vi "居中.vi"(8 "错误输入（无错误）":errorcluster, 11 "引用输入":refnum<vi>) -> (0 "错误输出":errorcluster, 3 "引用输出":refnum<vi>)   [LabVIEW 8.6, in "窗口操作.lvlib"]
doc: "<B>引用输入：</B>需要改变窗口的引用\n<B>引用输出：</B>需要改变窗口的引用输出\n\n编写者 ：曾嘉康\n编写时间：2014/12/12"
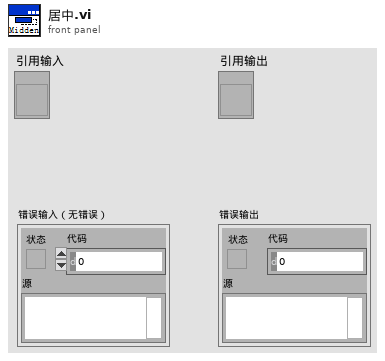
[diagram p1: front panel]
types:
  T1 = typedef "LVAllMonitorsDisplayTypeDef.ctl" = cluster{"Bounds":cluster{"Left":i16, "Top":i16, "Right":i16, "Bottom":i16}, "Depth":i16}[]
  T2 = typedef "LVRectTypeDef.ctl" = cluster{"Left":i16, "Top":i16, "Right":i16, "Bottom":i16}
  T3 = cluster{"Bounds":cluster{"Left":i16, "Top":i16, "Right":i16, "Bottom":i16}, "Depth":i16}
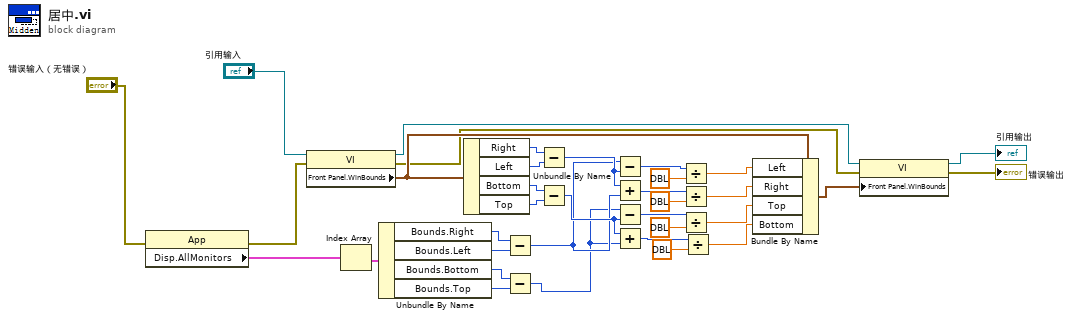
[diagram p0: block diagram]
diagram:
  n1 = property class="App"(error in="错误输入（无错误）") -> (error out=w24:errorcluster, "Disp.AllMonitors"=w34:T1)  [unwired: 1 in, 1 out]
  n2 = property class="VI"(reference="引用输入", error in=w24) -> (reference out=w15:refnum<vi>, error out=w18:errorcluster, "Front Panel.WinBounds"=w20:T2)
  n3 = Index Array ("索引数组")(array=w34) -> (element=w33:T3)  [unwired: 1 in]
  n4 = Unbundle By Name ("按名称解除捆绑")(w33) -> ("Bounds.Right"=w28:i16, "Bounds.Left"=w27:i16, "Bounds.Bottom"=w26:i16, "Bounds.Top"=w25:i16)
  n5 = Unbundle By Name(w20) -> ("Right"=w32:i16, "Left"=w29:i16, "Bottom"=w30:i16, "Top"=w31:i16)
  n6 = Subtract(x=w28, y=w27) -> (x-y=w2:i16)
  n7 = Subtract(x=w26, y=w25) -> (x-y=w1:i16)
  n8 = Subtract(x=w32, y=w29) -> (x-y=w22:i16)
  n9 = Subtract(x=w30, y=w31) -> (x-y=w21:i16)
  n10 = Subtract(x=w2, y=w22) -> (x-y=w14:i16)
  n11 = Add(x=w22, y=w2) -> (x+y=w13:i16)
  n12 = Subtract(x=w1, y=w21) -> (x-y=w12:i16)
  n13 = Add(x=w21, y=w1) -> (x+y=w11:i16)
  n14 = Divide(x=w14, y=dbl ?) -> (x/y=w7:dbl)
  n15 = Divide(x=w13, y=dbl ?) -> (x/y=w8:dbl)
  n16 = Divide(x=w12, y=dbl ?) -> (x/y=w10:dbl)
  n17 = Divide(x=w11, y=dbl ?) -> (x/y=w9:dbl)
  n18 = Bundle By Name(cluster=w20, "Left"=w7, "Right"=w8, "Top"=w10, "Bottom"=w9) -> (w19:T2)
  n19 = property class="VI"(reference=w15, error in=w18, "Front Panel.WinBounds"=w19) -> (reference out=→"引用输出":refnum<vi>, error out=→"错误输出":errorcluster)
